vi "Add Image to ImageList From ImageFile.vi"(8 "error in (no error)":errorcluster caption="错误输入（无错误）", 10 "Path":path, 11 "ImageListClass 输入":refnum<class "ImageListClass.lvclass"> caption="DNL_LabVIEW Object in") -> (0 "error out":errorcluster caption="错误输出", 3 "ImageListClass 输出":refnum<class "ImageListClass.lvclass"> caption="DNL_LabVIEW Object out")   [LabVIEW 2013, in "ImageListClass.lvclass"]
uses:
  ImageListClass.lvclass
  ImageListClass.lvclass/ImageListClass.ctl
  System.Drawing
  System.Windows.Forms
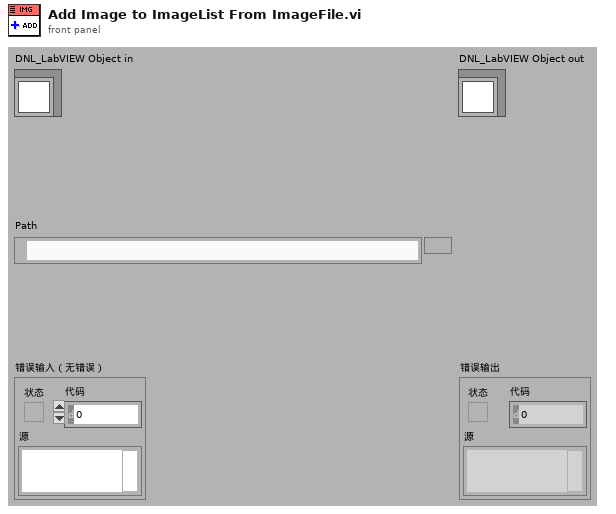
[diagram p1: front panel]
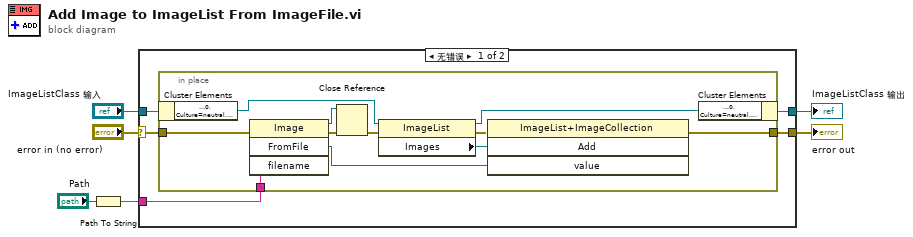
[diagram p0: block diagram]
diagram:
  n1 = Path To String(path="Path") -> (string=w1:string)
  n2 = case shown="无错误" "error in (no error)" {
    selector: "error in (no error)" -> [w10 w23]
    tunnel: [w8 w24] -> w4
    tunnel: "ImageListClass 输入" -> [w11 w24]
    tunnel: [w9 w23] -> w3
    tunnel: w1 -> [w7 _]
    frame No Error {
      n3 = in-place {
        in-place-border: w10 -> [w17]
        in-place-border: [w16] -> w9
        in-place-border: w7 -> [w15]
        n4 = in-place-cluster #1(w11) -> ("ImageList"=w22:refnum<k24>)
        n5 = invoke class="Image" method="FromFile"(error in=w17, "filename"=w15) -> (reference out=w13:refnum<k24>, error out=w14:errorcluster, "FromFile"=w20:refnum<k24>)  [unwired: 2 in, 1 out]
        n6 = Close Reference(reference=w13, error in (no error)=w14) -> (error out=w12:errorcluster)
        n7 = property class="ImageList"(reference=w22, error in=w12) -> (reference out=w19:refnum<k24>, error out=w18:errorcluster, "Images"=w21:refnum<k24>)
        n8 = invoke class="ImageList+ImageCollection" method="Add"(reference=w21, error in=w18, "value"=w20) -> (error out=w16:errorcluster)  [unwired: 1 in, 3 out]
        n9 = in-place-cluster #1("ImageList"=w19) -> (w8:refnum<class "ImageListClass.lvclass">)
      }
    }
    frame Error {
    }
  }
  "error out" <- w3
  "ImageListClass 输出" <- w4
